vi "Driver jsObject Array.vi"(8 "error in (no error)":errorcluster, 9 "DRIVERS (empty)":T1[](array[typedef]), 10 "Drivers jsObject Array Name (\"\")":string, 11 "Previous String (\"\")":string) -> (0 "error out":errorcluster, 3 "Drivers jsObject Array":string)   [LabVIEW 2011]
uses:
  Driver Record.ctl
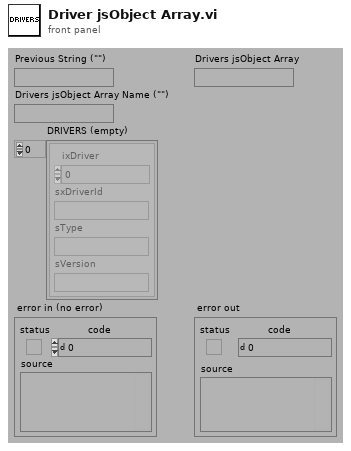
[diagram p1: front panel]
types:
  T1 = typedef "Driver Record.ctl" = cluster{"ixDriver":i32, "sxDriverId":string, "sType":string, "sVersion":string}
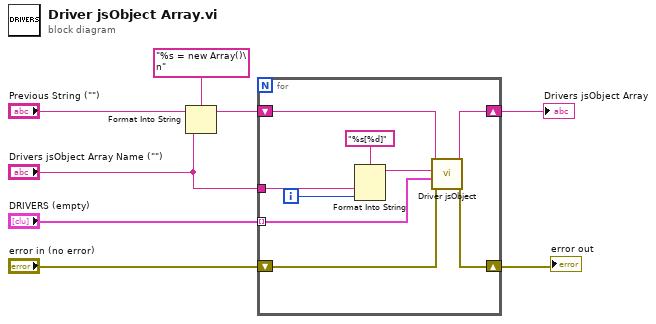
[diagram p0: block diagram]
diagram:
  n1 = Format Into String(format string="%s = new Array()\n", initial string="Previous String (\"\")", "Drivers jsObject Array Name (\"\")") -> (resulting string=w3:string)  [unwired: 1 in, 1 out]
  n2 = for {
    tunnel: "DRIVERS (empty)" -> [w16] mode=indexing
    shift-right: [w17] -> w7
    shift-left: w3 -> [w12]
    shift-right: [w15] -> w6
    shift-left: "error in (no error)" -> [w14]
    tunnel: "Drivers jsObject Array Name (\"\")" -> [w9]
    i -> [w10]
    n3 = Format Into String(format string="%s[%d]", w9, w10) -> (resulting string=w11:string)  [unwired: 2 in, 1 out]
    n4 = call "Driver jsObject.vi"("error in (no error)"=w14, "Station Record (empty)"=w16, "Driver jsObject Name (\"\")"=w11, "Previous String (\"\")"=w12) -> ("error out"=w15:errorcluster, "Driver jsObject"=w17:string)  [unwired: 6 out]
  }
  "Drivers jsObject Array" <- w7
  "error out" <- w6
